vi "Read Temperature.vi"(8 "error in (no error)":errorcluster) -> (0 "error IO":errorcluster, 1 "Array":dbl[](array[numeric]), 3 "decimal integer string":string[](array[string]))   [LabVIEW 2022 SP3]
doc: "Vi Used to read Temperature taken from the selected Moxa Channel\n-IoLogix E1262"
uses:
  <vilib>/NI/Modbus Library/API/Master/Modbus Master.lvclass
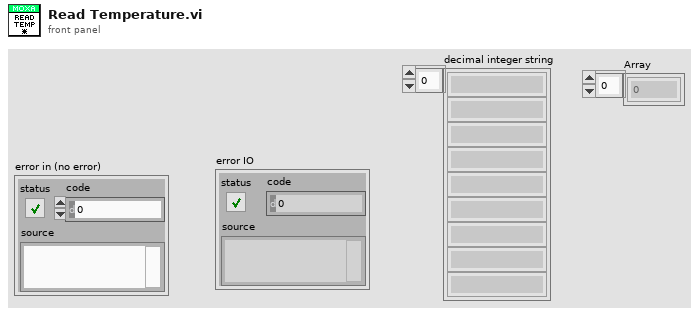
[diagram p1: front panel]
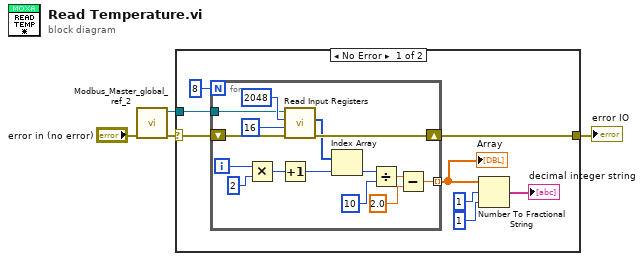
[diagram p0: block diagram]
diagram:
  n1 = call "Modbus_Master_global_ref_2.vi"("error in (no error) 2"="error in (no error)") -> ("error out 2"=w2:errorcluster, "Modbus Master out"=w3:refnum<class "Modbus Master.lvclass">)  [unwired: 9 in]
  n2 = case shown="No Error" w2 {
    selector: w2 -> [w10 w28]
    tunnel: [w12 w28] -> w4
    tunnel: w3 -> [w11 _]
    frame No Error {
      n3 = for {
        N: 8 -> [_]
        tunnel: [w16] -> w6 mode=indexing
        tunnel: w11 -> [w15]
        shift-right: [w25] -> w12
        shift-left: w10 -> [w14]
        i -> [w13]
        n4 = Multiply(x=w13, y=u8 2) -> (x*y=w20:i32)
        n5 = Increment(x=w20) -> (x+1=w19:i32)
        n6 = call-dynamic "Read Input Registers.vi"("error in"=w14, "number of inputs"=u16 16, "starting address"=u16 2048, "Modbus master in"=w15) -> ("error out"=w25:errorcluster, "register values"=w23:u16[])  [unwired: 5 in, 1 out]
        n7 = Index Array(array=w23, index=w19) -> (element=w22:u16)
        n8 = Divide(x=w22, y=u16 10) -> (x/y=w18:dbl)
        n9 = Subtract(x=w18, y=2.0) -> (x-y=w16:dbl)
      }
      "Array" <- w6
      n10 = Number To Fractional String(number=w6, width (-)=i16 1, precision (6)=i16 1 ("width (-)")) -> (F-format string=→"decimal integer string":string[])  [unwired: 1 in]
    }
    frame Error {
    }
  }
  "error IO" <- w4
